vi "Cycling.vi"() -> ()   [LabVIEW 2020]
panel:
  in  "Current Cutoff":dbl
  in  "Number of Cycles":i32
  in  "Charge filepath":path
  in  "Discharge filepath":path
  in  "Batteryname":string
  in  "Starting Cycle":i32
  out "PS error out":errorcluster
  out "PS Visa Out":refnum<visa-resource-name>
  out "parallel task error out":errorcluster
  out "parallel task out":refnum<k21>
  in  "Wait time":dbl
  in  "Discharge Current Setpoint":dbl format="%#.6g"
  in  "Charge Current Setpoint":dbl format="%#.6g"
  in  "Battery Type":enum16{"30Q", "40T", "Nissan Leaf"}(ring)
  in  "PS type":enum16{"NHR", "ITECH"}(ring)
  in  "#DAQ outputs (1-13)":i32
  in  "Data Task in":refnum<k21>
  in  "data task error in":errorcluster
  in  "PS error in":errorcluster caption="PS error in (no error)"
  in  "PS VISA in":refnum<visa-resource-name>
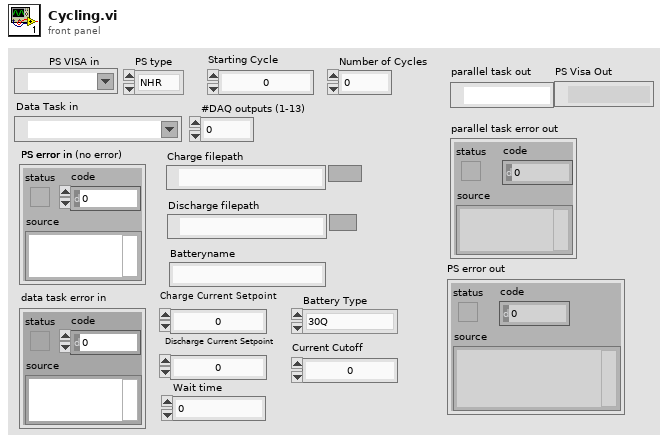
[diagram p1: front panel]
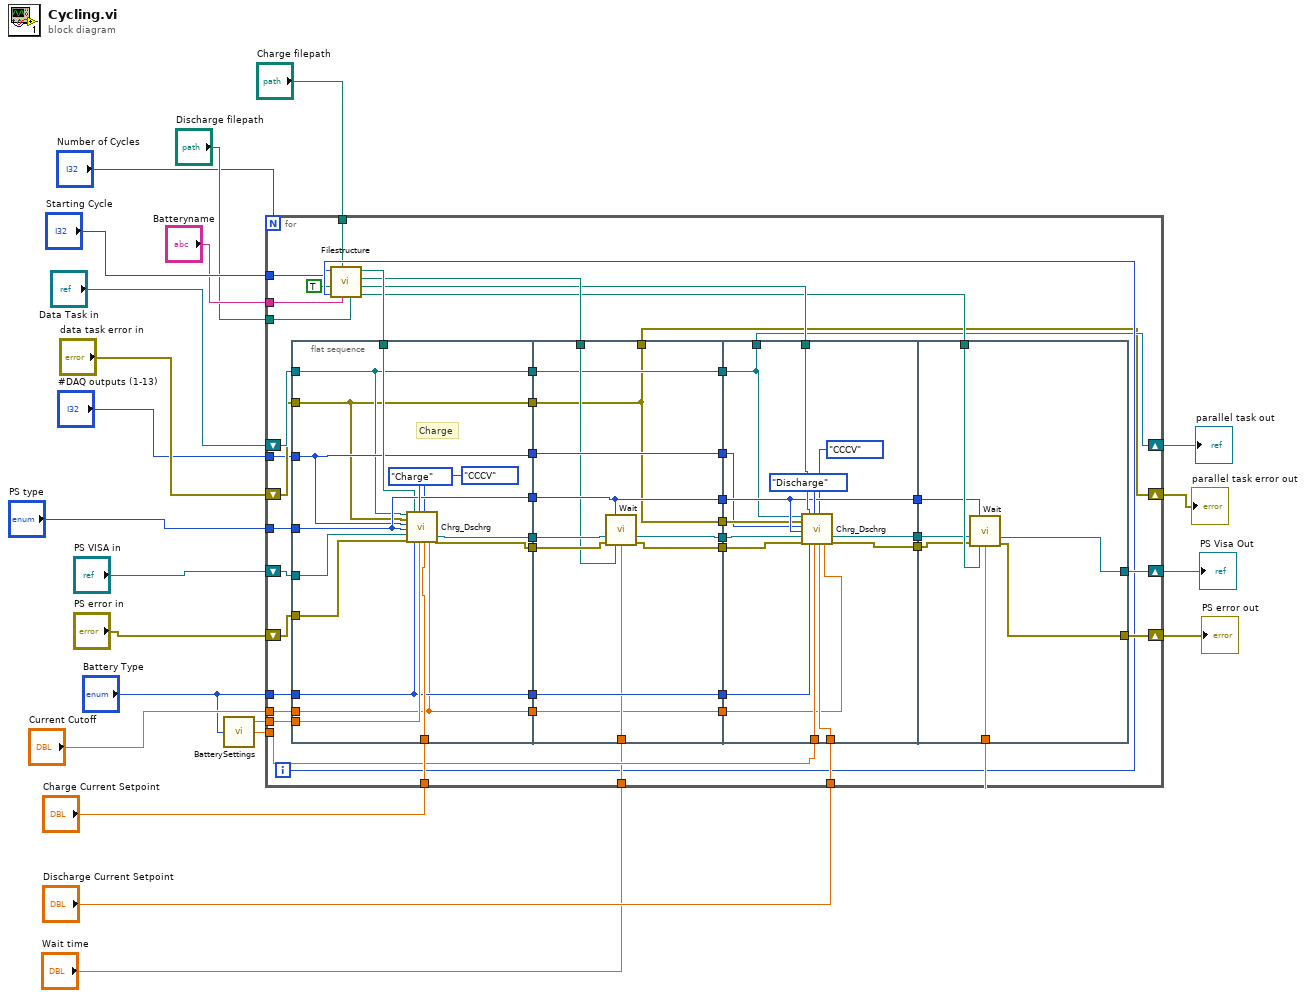
[diagram p0: block diagram]
diagram:
  n1 = call "BatterySettings.vi"("Battery Type"="Battery Type") -> ("Min Voltage (V)"=w14:dbl, "Max Voltage (V)"=w16:dbl)  [unwired: 2 in, 1 out]
  n2 = for {
    N: "Number of Cycles" -> [_]
    tunnel: "#DAQ outputs (1-13)" -> [w53]
    tunnel: "PS type" -> [w52]
    tunnel: w16 -> [w49]
    tunnel: "Battery Type" -> [w48]
    tunnel: "Charge Current Setpoint" -> [w47]
    tunnel: w14 -> [w46]
    tunnel: "Discharge Current Setpoint" -> [w45]
    tunnel: "Wait time" -> [w40]
    shift-right: [w27] -> w8
    shift-left: "Data Task in" -> [w55]
    shift-right: [w26] -> w9
    shift-left: "data task error in" -> [w54]
    shift-right: [w38] -> w10
    shift-left: "PS VISA in" -> [w51]
    shift-right: [w39] -> w11
    shift-left: "PS error in" -> [w50]
    tunnel: "Starting Cycle" -> [w36]
    tunnel: "Batteryname" -> [w34]
    tunnel: "Discharge filepath" -> [w33]
    tunnel: "Charge filepath" -> [w32]
    tunnel: "Current Cutoff" -> [w25]
    i -> [w37]
    n3 = flat-sequence {
      tunnel: w55 -> [w72]
      tunnel: w54 -> [w71]
      tunnel: w53 -> [w73]
      tunnel: w52 -> [w76]
      tunnel: w51 -> [w83]
      tunnel: w50 -> [w82]
      tunnel: w48 -> [w75]
      tunnel: w49 -> [w80]
      tunnel: w47 -> [w79]
      tunnel: [w78] -> w68
      tunnel: [w77] -> w67
      tunnel: [w76] -> w66
      tunnel: [w73] -> w65
      tunnel: [w75] -> w64
      tunnel: w44 -> [w74]
      tunnel: [w72] -> w31
      tunnel: [w71] -> w29
      tunnel: w25 -> [w69]
      tunnel: [w69] -> w24
      tunnel: w68 -> [w95]
      tunnel: w67 -> [w94]
      tunnel: w66 -> [w90]
      tunnel: [w93] -> w63
      tunnel: [w92] -> w62
      tunnel: w65 -> [w91]
      tunnel: [w91] -> w61
      tunnel: [w90] -> w60
      tunnel: w64 -> [w89]
      tunnel: [w89] -> w59
      tunnel: w43 -> [w88]
      tunnel: w40 -> [w87]
      tunnel: w31 -> [w86]
      tunnel: [w86] -> w30
      tunnel: w29 -> [w85]
      tunnel: [w85] -> w28
      tunnel: [w85] -> w26
      tunnel: w24 -> [w84]
      tunnel: [w84] -> w23
      tunnel: w63 -> [w110]
      tunnel: w62 -> [w109]
      tunnel: w61 -> [w99]
      tunnel: w60 -> [w101]
      tunnel: w59 -> [w108]
      tunnel: w46 -> [w107]
      tunnel: w45 -> [w106]
      tunnel: w42 -> [w104]
      tunnel: [w103] -> w58
      tunnel: [w102] -> w57
      tunnel: [w101] -> w56
      tunnel: w30 -> [w98]
      tunnel: w28 -> [w100]
      tunnel: [w98] -> w27
      tunnel: w23 -> [w96]
      tunnel: w41 -> [w117]
      tunnel: w58 -> [w116]
      tunnel: w57 -> [w115]
      tunnel: w40 -> [w114]
      tunnel: w56 -> [w113]
      tunnel: [w112] -> w39
      tunnel: [w111] -> w38
      frame #0 {
        # "Charge"
        n4 = call "Chrg_Dschrg.vi"("Data Task in"=w72, "data task error in"=w71, "#DAQ outputs (1-13)"=w73, "PS type"=w76, "PS VISA in"=w83, "PS error in"=w82, "DischargeCyclePath"=w74, "Battery Type"=w75, "Charge/discharge"=enum8{"Charge", "Discharge"}."Charge", "Charge/Discharge Voltage Setpoint"=w80, "CC or CCCV"=enum16{"CC", "CCCV"}."CCCV", "Current Setpoint"=w79, "Current Cutoff"=w69) -> ("PS VIS resource name out"=w78:refnum<visa-resource-name>, "PS error out"=w77:errorcluster)  [unwired: 3 in, 2 out]
      }
      frame #1 {
        n5 = call "Wait.vi"("PS type"=w90, "PS VISA in"=w95, "PS error in"=w94, "Wait Filepath"=w88, "Wait time"=w87) -> ("PS Visa Out"=w93:refnum<visa-resource-name>, "PS error out"=w92:errorcluster)  [unwired: 7 in, 2 out]
      }
      frame #2 {
        n6 = call "Chrg_Dschrg.vi"("Data Task in"=w98, "data task error in"=w100, "#DAQ outputs (1-13)"=w99, "PS type"=w101, "PS VISA in"=w110, "PS error in"=w109, "DischargeCyclePath"=w104, "Battery Type"=w108, "Charge/discharge"=enum8{"Charge", "Discharge"}."Discharge", "Charge/Discharge Voltage Setpoint"=w107, "CC or CCCV"=enum16{"CC", "CCCV"}."CCCV", "Current Setpoint"=w106, "Current Cutoff"=w96) -> ("PS VIS resource name out"=w103:refnum<visa-resource-name>, "PS error out"=w102:errorcluster)  [unwired: 3 in, 2 out]
      }
      frame #3 {
        n7 = call "Wait.vi"("PS type"=w113, "PS VISA in"=w116, "PS error in"=w115, "Wait Filepath"=w117, "Wait time"=w114) -> ("PS Visa Out"=w111:refnum<visa-resource-name>, "PS error out"=w112:errorcluster)  [unwired: 7 in, 2 out]
      }
    }
    n8 = call "Filestructure.vi"("Discharge filepath"=w33, "Batteryname"=w34, "Charge filepath"=w32, "For loop i"=w37, "In for loop"=TRUE, "Starting Cycle"=w36) -> ("DischargeWaitPath"=w41:path, "DischargeCyclePath"=w42:path, "ChargeWaitPath"=w43:path, "ChargeCyclePath"=w44:path)  [unwired: 1 in, 1 out]
  }
  "PS error out" <- w11
  "PS Visa Out" <- w10
  "parallel task error out" <- w9
  "parallel task out" <- w8
